vi "DMM6500.vi"(8 "error in (no error)":errorcluster) -> (0 "error in (out)":errorcluster)   [LabVIEW 2024, in "DMM6500.lvlib"]
doc: "This template is for the Queued Message Handler design pattern.\n\nThe Event Handling Loop generates messages based on user interface actions.\n\nThe Message Handling Loop processes messages generated by the Event Handling Loop, or by other messages. The messages are string values, so new messages can be added easily to the Message Cases case structure in the Message Handling Loop. Each message cluster can also provide an optional value for Message Data, which is a variant that can be converted to whatever message-specific data is required."
uses:
  DMM6500.lvlib
  controls/DMM6500 UI Data.ctl
  Settings/support/DAQ_Config.ctl
  PrivateControls/DMM6500_FGV_Queue_Control.ctl
  687c9c7c-8178-403c-bf7e-b93dd3f91936.vi
  21044260-a770-49ae-a215-1be9417de303.vi
  <instrlib>/Keithley DMM6500 DAQ6500 Series/Public/Data/Read (Multiple Points).vi
  <vilib>/Utility/error.llb/Error Cluster From Error Code.vi
  <vilib>/ErrorRing/Error Ring.xnode
  support/Message Queue/DMM6500 Message Queue.lvlib
  support/User Event - Stop/DMM6500 User Event - Stop.lvlib
  <instrlib>/Keithley DMM6500 DAQ6500 Series/Keithley DMM6500 DAQ6500 Series.lvlib
  Launcher/Launcher_DTU.lvlib
  Settings/Setting_Screen.lvlib
  <instrlib>/Keithley DMM6500 DAQ6500 Series/Public/Data/Read (Single Point).vi
panel:
  out "status":bool
  in  "Scan Count (2)":u32=5
  in  "Config":string
  in  "DUT":string
  in  "Scan Count (1)":u32=5
  in  "DMM6500":refnum<visa-resource-name>="USB0::0x05E6::0x6510::04596852::INSTR"
  out "Data":dbl[](array[numeric])
  in  "Channel List(\"\")":string
  in  "Function":i32(ring) items=["Voltage DC", "Voltage AC", "Current DC", "Current AC", "Resistance", "4-wire Resistance", "Diode", "Capacitance", "Temperature", "Continuity", "Frequency", "Period", "Voltage Ratio", "Digitize Voltage", "Digitize Current"]
  out "queue name 2":string
  out "queue name":string
  out "Display <Replace Me>":string
  in  "Measure":bool
  in  "Do Something <Replace Me>":bool
  in  "Exit":bool
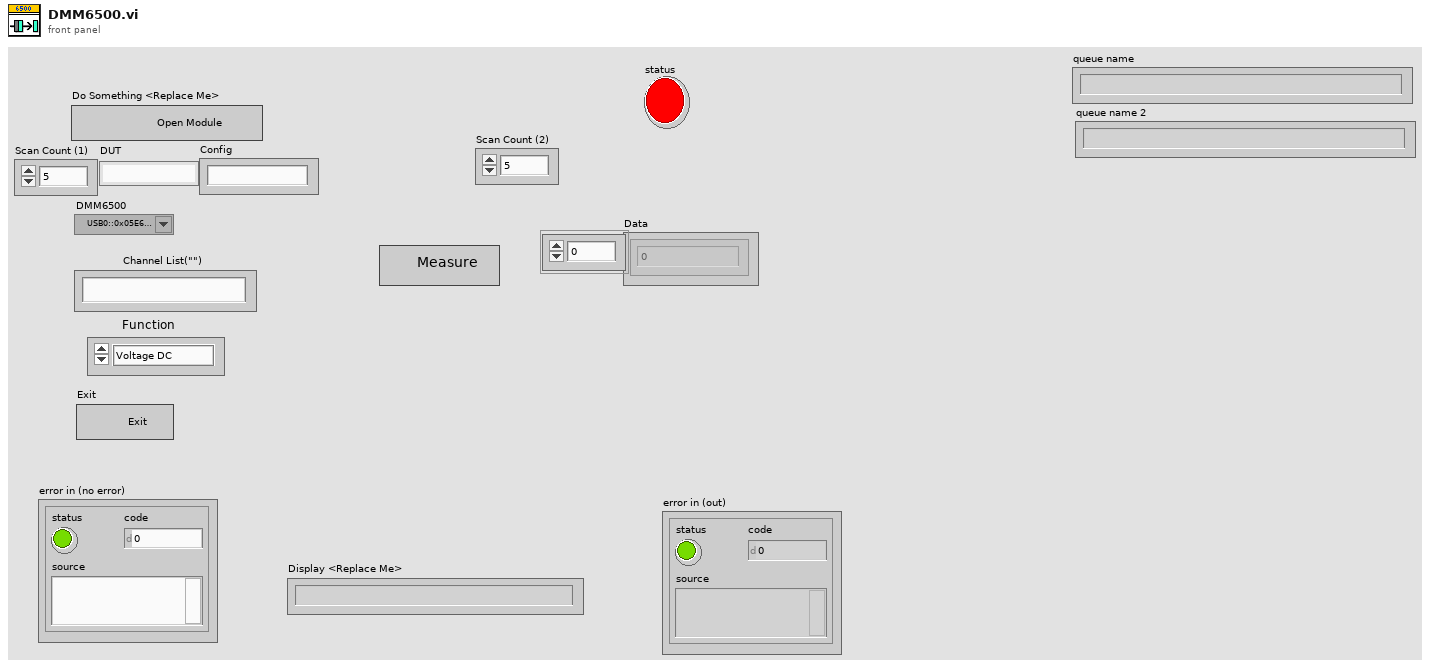
[diagram p1: front panel]
types:
  T1 = typedef "DMM6500.lvlib/DMM6500 UI Data.ctl" = cluster{"Config":string, "VISA":refnum<visa-resource-name>, "Function":i32, "Channel List(\"\")":string, "VISA resource name":refnum<visa-resource-name>, "Pseudo Card (0:No pseudocard)":i32, "Slot Number (0: slot1)":i32, "queue in":refnum<queue>, "DUT":string, "notifier out":refnum<notifier>}
  T2 = typedef "DMM6500.lvlib/DMM6500_FGV_Queue_Control.ctl" = enum16{"Release", "Get", "Set"}
  T3 = typedef "DMM6500.lvlib/DMM6500 Message Queue.lvlib/DMM6500_All Message Queues.ctl" = cluster{"UI":refnum<queue>, "QSM":refnum<queue>}
  T4 = cluster{"Message":string, "Message Data":variant}
  T5 = cluster{"Baud Rate":u32, "Flow Control":u16, "Parity":u16, "Stop Bits":u16, "Data Bits":u16}
  T6 = enum16{"Read", "Write", "All_sections", "All_values", "Remove key&section"}
  T7 = typedef "Setting_Screen.lvlib/DAQ_Config.ctl" = cluster{"AUTO RANGE":bool, "CHANNEL LIST":string, "SELECT Card":u16, "SELECT SLOT":u16, "Function":i32}
  T8 = cluster{"Function":i32, "Channel List(\"\")":string}
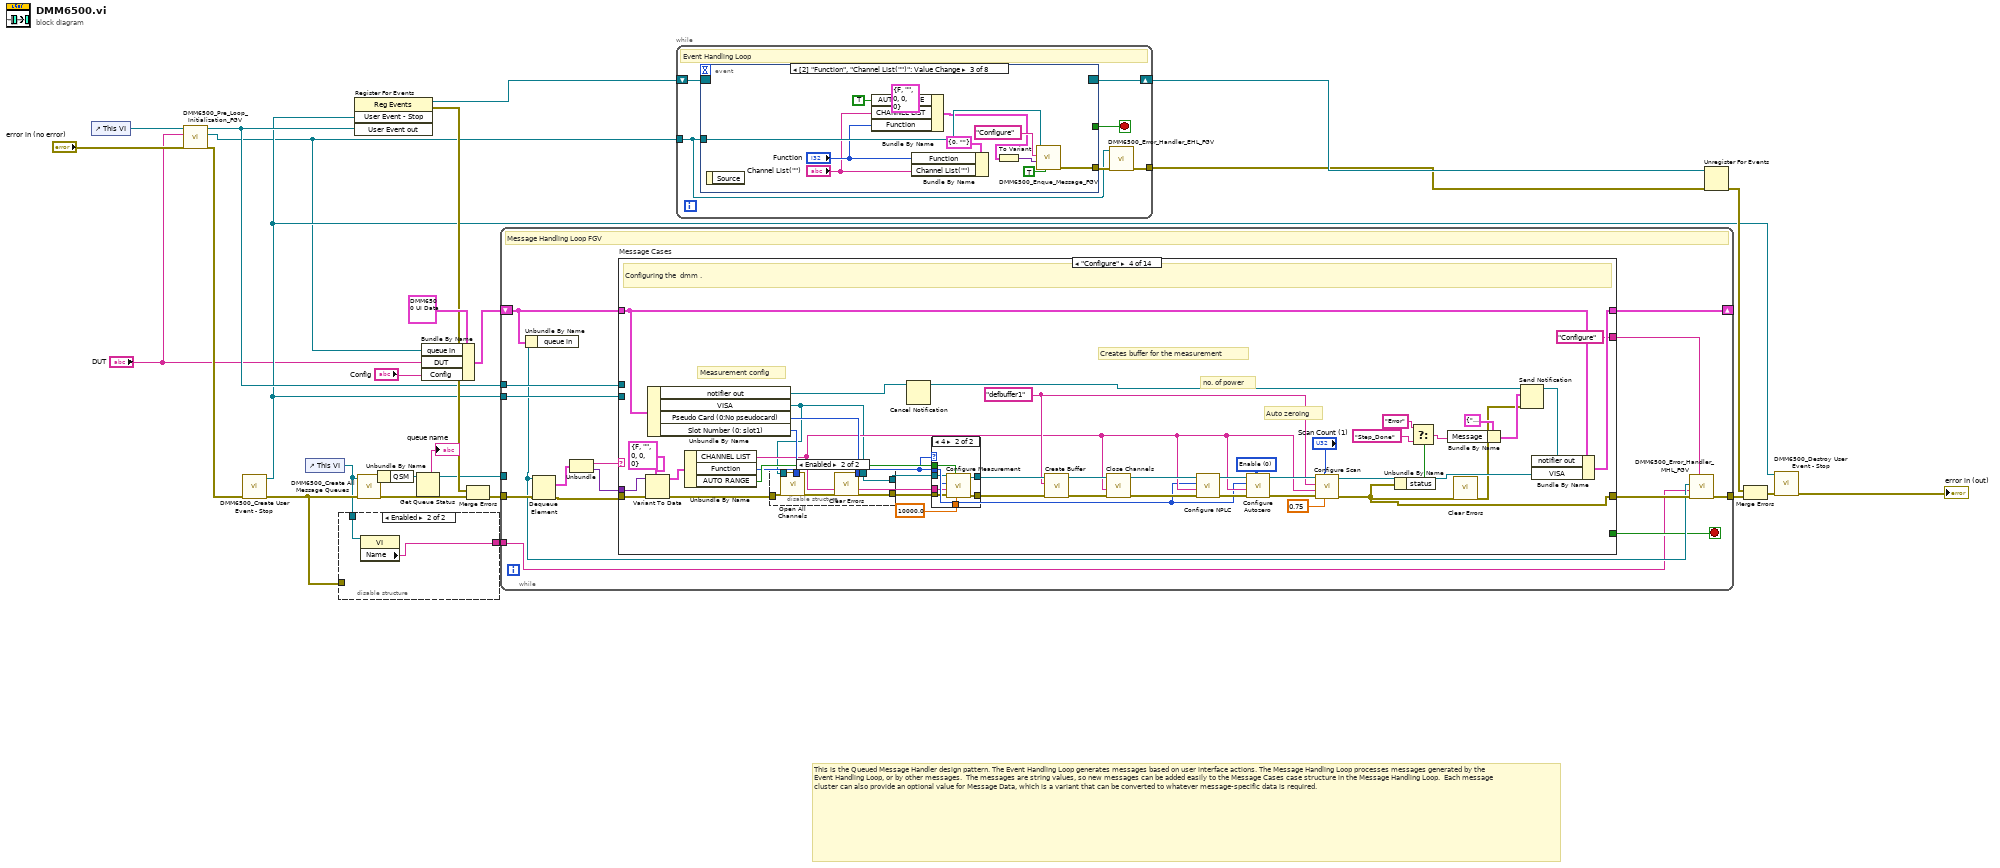
[diagram p0: block diagram]
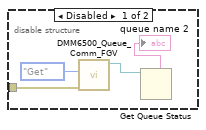
[diagram p2: hidden frame]
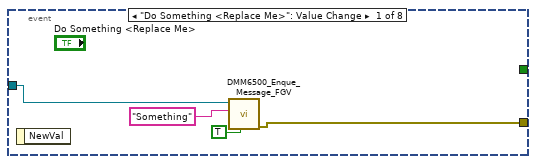
[diagram p3: hidden frame]
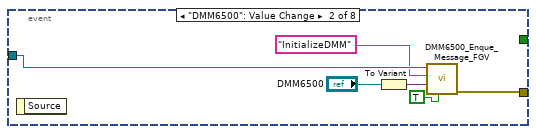
[diagram p4: hidden frame]
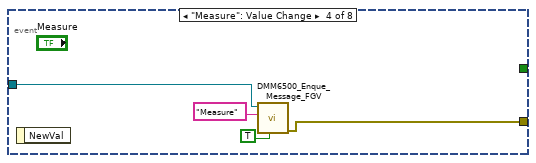
[diagram p5: hidden frame]
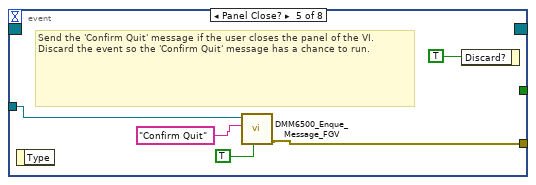
[diagram p6: hidden frame]
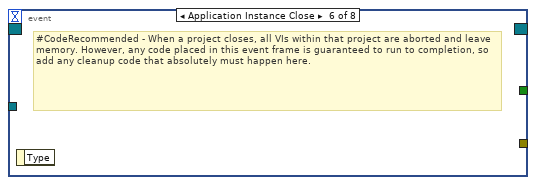
[diagram p7: hidden frame]
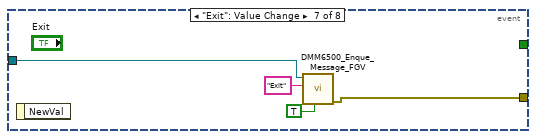
[diagram p8: hidden frame]
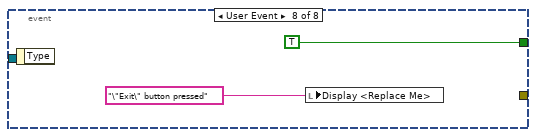
[diagram p9: hidden frame]
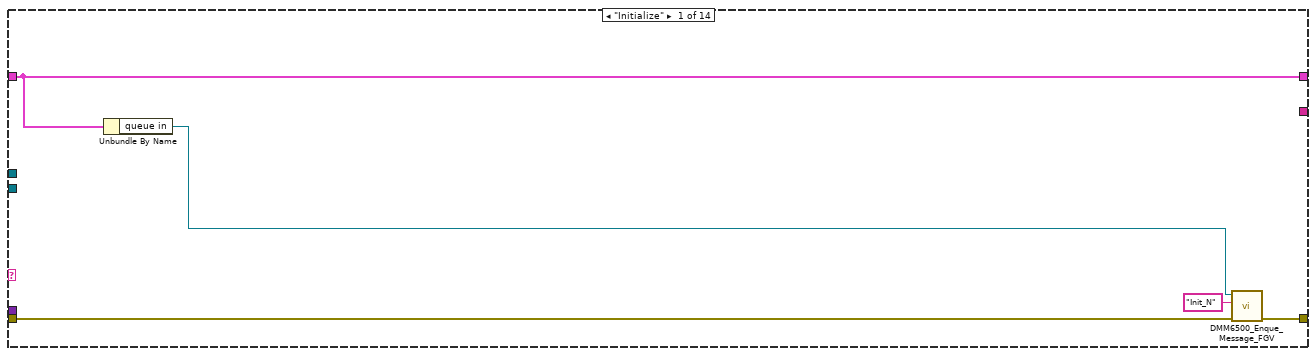
[diagram p10: hidden frame]
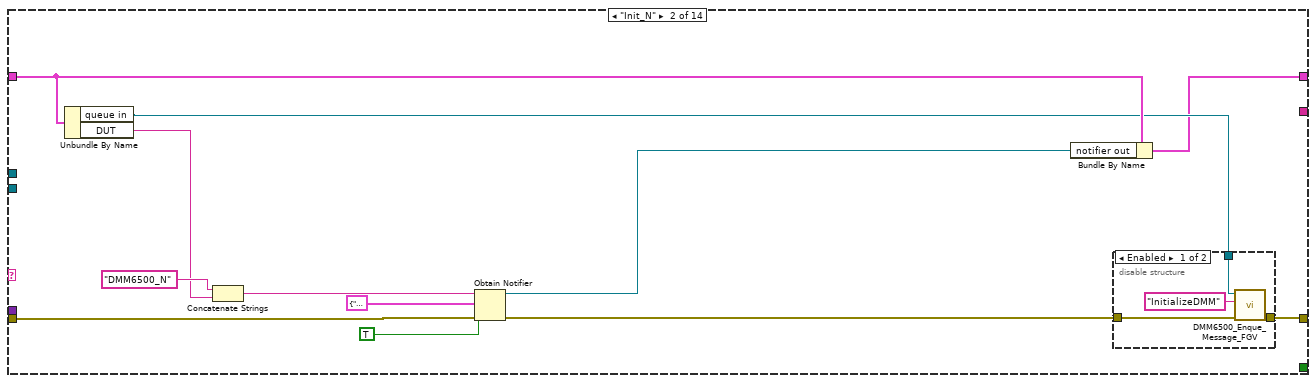
[diagram p11: hidden frame]
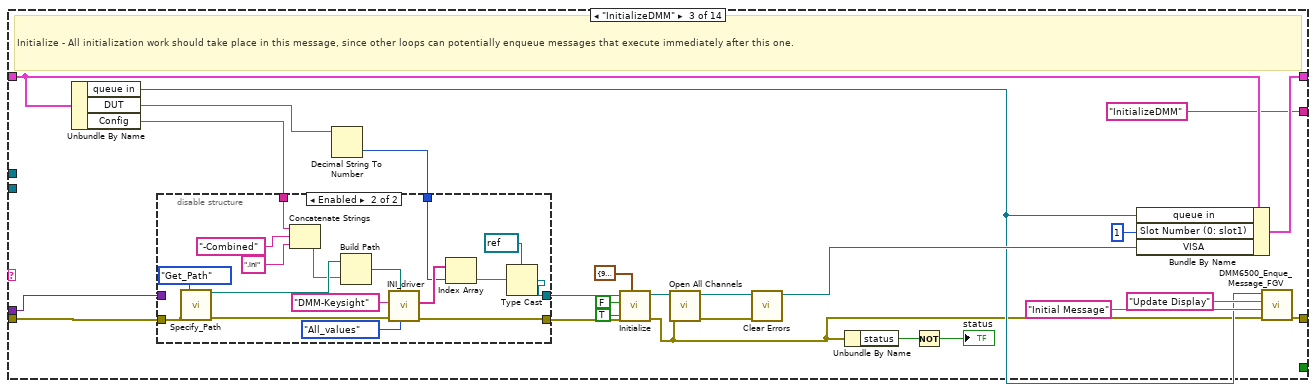
[diagram p13: hidden frame]
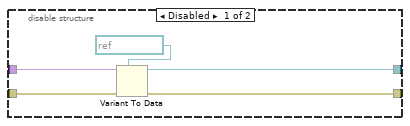
[diagram p14: hidden frame]
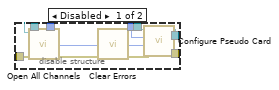
[diagram p15: hidden frame]
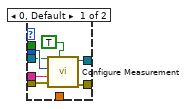
[diagram p16: hidden frame]
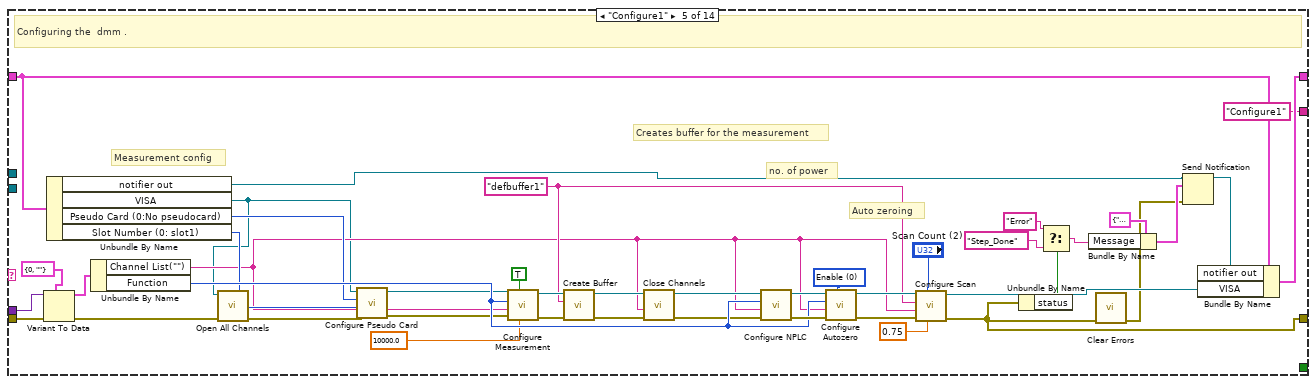
[diagram p17: hidden frame]
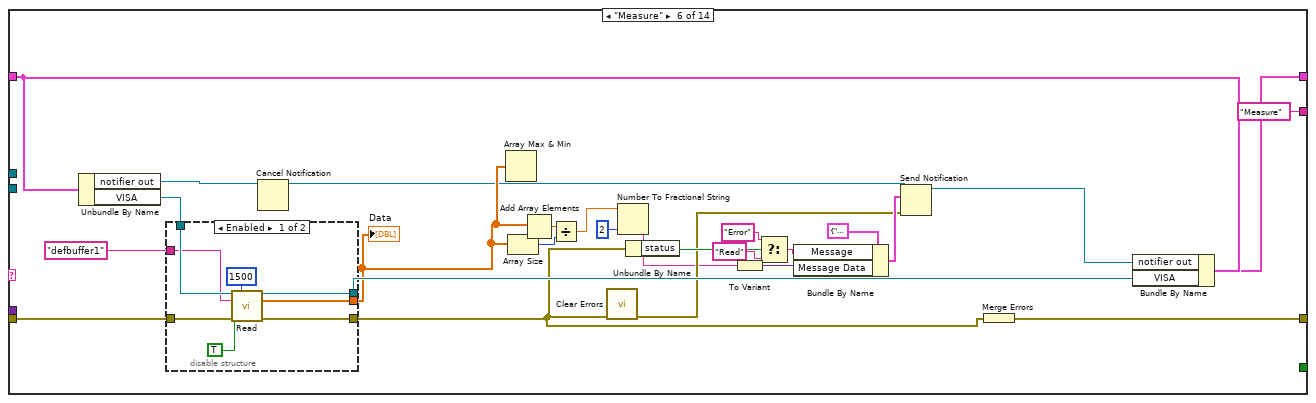
[diagram p18: hidden frame]
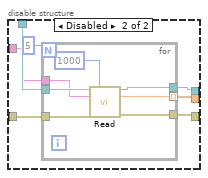
[diagram p19: hidden frame]
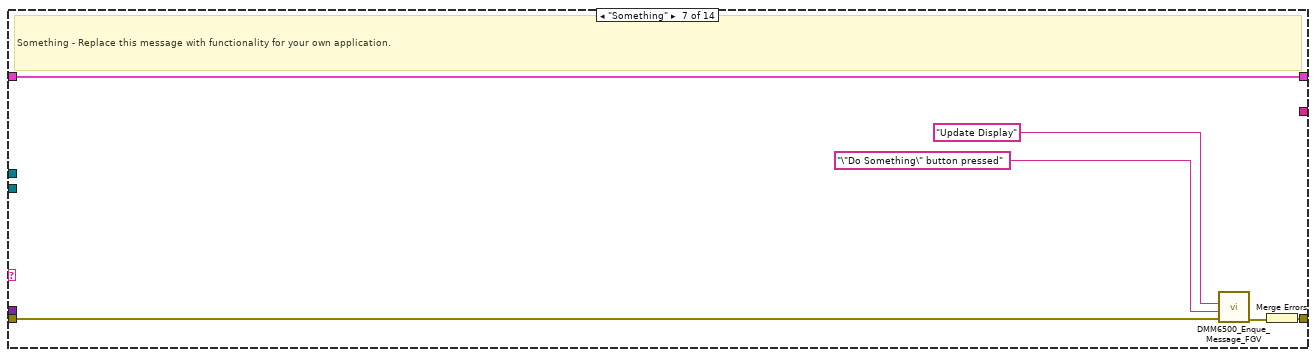
[diagram p20: hidden frame]
diagram:
  # "This is the Queued Message Handler design pattern. The Event Handling Loop generates messages based on user interface actions. The Message Handling Loop processes messages generated by the Event Handling Loop, or by other messages.  The messages are string values, so new messages can be added easily to the Message Cases case structure in the Message Handling Loop.  Each message cluster can also provide an optional value for Message Data, which is a variant that can be converted to whatever message-specific data is required."
  n1 = control-ref of="This VI"() -> (w15:refnum<vi>)
  n2 = call "DMM6500_Pre_Loop_Initialization_FGV.vi"("error in (no error)"="error in (no error)", "DUT"="DUT", "VI in"=w15) -> ("error out"=w13:errorcluster, "queue out"=w5:refnum<queue>, "User Event out"=w8:refnum<user-event>)  [unwired: 6 in]
  n3 = call "DMM6500_Create User Event - Stop.vi"("error in (no error)"=w13) -> ("error out"=w9:errorcluster, "User Event - Stop"=w7:refnum<user-event>)  [unwired: 9 in]
  n4 = control-ref of="This VI"() -> (w2:refnum<vi>)
  n5 = disable-structure shown="Enabled" {
    disable-tunnel: w9 -> [w31 _]
    disable-tunnel: w2 -> [_ w33]
    disable-tunnel: [_ w32] -> w1
    frame Disabled {
      n6 = call "DMM6500_Queue_Comm_FGV.vi"("error in (no error)"=w31, "Enum"=DMM6500_FGV_Queue_Control."Get") -> ("queue Out"=w29:refnum<queue>)  [unwired: 8 in, 1 out]
      n7 = Get Queue Status(queue=w29) -> (queue name=→"queue name 2":string)  [unwired: 2 in, 7 out]
    }
    frame Enabled {
      n8 = property class="VI"(reference=w33) -> ("Name"=w32:string)  [unwired: 1 in, 2 out]
    }
  }
  n9 = register-events(w7, w8) -> (reference out=w18:refnum<event-registration>, error out=w16:errorcluster)  [unwired: 2 in]
  n10 = call "DMM6500_Create All Message Queues.vi"("error in (no error)"=w9, "This VI"=w2) -> ("error out"=w27:errorcluster, "Message Queues out"=w26:T3)  [unwired: 8 in]
  n11 = Unbundle By Name(w26) -> ("QSM"=w24:refnum<queue>)
  n12 = Get Queue Status(queue=w24) -> (queue out=w11:refnum<queue>, queue name=→"queue name":string)  [unwired: 2 in, 6 out]
  n13 = Bundle By Name(cluster=T1 {"Config"="", "VISA"="", "Function"=0, "Channel List(\"\")"="", "VISA resource name"="USB0::0x05E6::0x6510::04596852::INSTR", "Pseudo Card (0:No pseudocard)"=0, "Slot Number (0: slot1)"=0, "queue in"=refnum, "DUT"="", "notifier out"=refnum} ("Data Cluster"), "queue in"=w5, "DUT"="DUT", "Config"="Config") -> (w6:T1)
  n14 = Merge Errors(w16, w27) -> (w17:errorcluster)
  n15 = while {
    tunnel: w11 -> [_]
    shift-right: [w48] -> _
    shift-left: w6 -> [w41]
    tunnel: w8 -> [w47]
    tunnel: w17 -> [w43]
    tunnel: [w45] -> w25
    tunnel: w7 -> [w44]
    tunnel: w1 -> [w35]
    stop <- w36 stop-if-true
    # "Message Handling Loop FGV"
    n16 = Unbundle By Name(w41) -> ("queue in"=w37:refnum<queue>)
    n17 = Dequeue Element(queue=w37, error in (no error)=w43) -> (element=w40:T4, error out=w42:errorcluster)  [unwired: 1 in, 2 out]
    n18 = Unbundle(w40) -> ("Message"=w39:string, "Message Data"=w38:variant)
    n19 = case "Message Cases" shown="\"Configure\"" w39 {
      selector: w39 -> [_ _ _ _ _ _ _ _ _ _ _ _ _ w363]
      tunnel: w42 -> [w53 w58 w83 w145 w215 w256 w279 w285 w295 w311 w326 w345 w358 _]
      tunnel: [w52 w65 w93 w120 w189 w242 w283 w289 w296 w300 w316 w347 w349 w364] -> w46
      tunnel: w41 -> [w50 w64 w90 w159 w230 w255 w284 w290 w297 w309 w322 w342 w353 w365]
      tunnel: [w50 w55 w94 w148 w218 w252 w284 w290 w297 w309 w322 w342 w353 w365] -> w48
      tunnel: [_ _ _ _ _ _ _ _ _ _ _ _ TRUE _] -> w36
      tunnel: w38 -> [_ _ w84 w146 w216 _ _ _ w294 _ w325 _ _ _]
      tunnel: w47 -> [_ _ _ _ _ _ _ _ _ _ _ _ w360 _]
      tunnel: w44 -> [_ _ _ _ _ _ _ _ _ _ _ _ w356 _]
      tunnel: [_ _ "InitializeDMM" "Configure" "Configure1" "Measure" _ _ _ _ "Error" _ _ _] -> w34
      frame "Initialize" {
        n20 = Unbundle By Name(w50) -> ("queue in"=w49:refnum<queue>)
        n21 = call "DMM6500_Enque_Message_FGV.vi"("error in (no error)"=w53, "Message"="Init_N", "queue In"=w49) -> ("error out"=w52:errorcluster)  [unwired: 8 in]
      }
      frame "Init_N" {
        n22 = Unbundle By Name(w64) -> ("queue in"=w63:refnum<queue>, "DUT"=w56:string)
        n23 = Concatenate Strings("DMM6500_N", w56) -> (w61:string)
        n24 = Obtain Notifier(name (unnamed)=w61, notification data type=T4 {"Message"="", "Message Data"=variant} ("notification"), create if not found? (T)=TRUE, error in (no error)=w58) -> (notifier out=w54:refnum<notifier>, error out=w57:errorcluster)  [unwired: 1 out]
        n25 = Bundle By Name(cluster=w64, "notifier out"=w54) -> (w55:T1)
        n26 = disable-structure shown="Enabled" {
          disable-tunnel: [w68 w70] -> w65
          disable-tunnel: w63 -> [w67 _]
          disable-tunnel: w57 -> [w66 w70]
          frame Enabled {
            n27 = call "DMM6500_Enque_Message_FGV.vi"("error in (no error)"=w66, "Message"="InitializeDMM", "queue In"=w67) -> ("error out"=w68:errorcluster)  [unwired: 8 in]
          }
          frame Disabled {
          }
        }
      }
      frame "InitializeDMM" {
        # "Initialize - All initialization work should take place in this message, since other loops can potentially enqueue messages that execute immediately after this one."
        n28 = Unbundle By Name(w90) -> ("queue in"=w86:refnum<queue>, "DUT"=w81:string, "Config"=w85:string)
        n29 = Decimal String To Number(string=w81) -> (number=w80:i32)  [unwired: 2 in, 1 out]
        n30 = disable-structure shown="Enabled" {
          disable-tunnel: w83 -> [w99 w104]
          disable-tunnel: [w98 w102] -> w82
          disable-tunnel: w84 -> [w97 _]
          disable-tunnel: [w95 w103] -> w79
          disable-tunnel: w85 -> [_ w101]
          disable-tunnel: w80 -> [_ w100]
          frame Disabled {
            n31 = Variant To Data(error in=w99, type=refnum<visa-resource-name> "COM27" ("VISA resource name"), Variant=w97) -> (data=w95:refnum<visa-resource-name>, error out=w98:errorcluster)
          }
          frame Enabled {
            n32 = call "Specify_Path.vi"("Path_Enum"=enum16{"Find_Path", "Get_Path"}."Get_Path", "error in (no error)"=w104) -> ("Configurations"=w113:path, "error out"=w109:errorcluster)  [unwired: 6 in, 6 out]
            n33 = Concatenate Strings(w101, "-Combined" ("string"), ".ini" ("string")) -> (w112:string)
            n34 = Build Path(base path=w113, name or relative path=w112) -> (appended path=w111:path)
            n35 = call "INI_driver.vi"("Enum"=T6."All_values", "instrument file path"=w111, "error in (no error)"=w109, "Section"="DMM-Keysight") -> ("error out"=w102:errorcluster, "Values out"=w107:string[])  [unwired: 4 in, 2 out]
            n36 = Index Array(array=w107, index=w100) -> (element=w106:string)
            n37 = Type Cast(type=refnum<visa-resource-name> refnum ("VISA resource name"), x=w106) -> (*(type *) &x=w103:refnum<visa-resource-name>)
          }
        }
        n38 = call <instrlib>:"Initialize.vi"("Serial Configuration"=T5 {"Baud Rate"=9600, "Flow Control"=0, "Parity"=0, "Stop Bits"=10, "Data Bits"=8}, "error in (no error)"=w82, "Reset (True)"=TRUE, "ID Query (True)"=FALSE, "VISA resource name"=w79) -> ("error out"=w71:errorcluster, "VISA resource name out"=w88:refnum<visa-resource-name>)  [unwired: 5 in]
        n39 = call <instrlib>:"Open All Channels.vi"("error in (no error)"=w71, "VISA resource name"=w88) -> ("error out"=w74:errorcluster, "VISA resource name out"=w87:refnum<visa-resource-name>)  [unwired: 8 in]
        n40 = call <vilib>:"Clear Errors.vi"("error in (no error)"=w74) -> ()  [unwired: 5 in, 2 out]
        n41 = Unbundle By Name(w71) -> ("status"=w73:bool)
        n42 = Not(x=w73) -> (.not. x?=→"status":bool)
        n43 = Bundle By Name(cluster=w90, "queue in"=w86, "Slot Number (0: slot1)"=1, "VISA"=w87) -> (w94:T1)
        n44 = call "DMM6500_Enque_Message_FGV.vi"("error in (no error)"=w71, "Message Data"="Initial Message" ("Initial Message"), "Message"="Update Display", "queue In"=w86) -> ("error out"=w93:errorcluster)  [unwired: 7 in]
      }
      frame "Configure" {
        w151 = u32 0 items=["Enable", "Disable", "Once"] ("Auto Zero (0: Enable)")
        w150 = "defbuffer1" ("Buffer Name (\"\")")
        # "Auto zeroing"
        # "no. of power"
        # "Creates buffer for the measurement"
        # "Measurement config"
        # "Configuring the  dmm ."
        n45 = Variant To Data(error in=w145, type=T7 {"AUTO RANGE"=FALSE, "CHANNEL LIST"="", "SELECT Card"=0, "SELECT SLOT"=0, "Function"=0} ("DAQ_Config"), Variant=w146) -> (data=w144:T7, error out=w143:errorcluster)
        n46 = Unbundle By Name(w159) -> ("notifier out"=w128:refnum<notifier>, "VISA"=w118:refnum<visa-resource-name>, "Pseudo Card (0:No pseudocard)"=w141:i32, "Slot Number (0: slot1)"=w140:i32)
        n47 = Unbundle By Name(w144) -> ("CHANNEL LIST"=w135:string, "Function"=w121:i32, "AUTO RANGE"=w122:bool)
        n48 = disable-structure shown="Enabled" {
          disable-tunnel: w143 -> [w167 w171]
          disable-tunnel: [w166 w172] -> w142
          disable-tunnel: w141 -> [w165 _]
          disable-tunnel: w140 -> [w164 _]
          disable-tunnel: [w163 w168] -> w139
          disable-tunnel: w118 -> [w161 w172]
          disable-tunnel: w118 -> [_ w169]
          frame Disabled {
            n49 = call <instrlib>:"Open All Channels.vi"("error in (no error)"=w167, "VISA resource name"=w161) -> ("error out"=w162:errorcluster)  [unwired: 8 in, 1 out]
            n50 = call <vilib>:"Clear Errors.vi"("error in (no error)"=w162) -> ("error out"=w160:errorcluster)  [unwired: 5 in, 1 out]
            n51 = call <instrlib>:"Configure Pseudo Card.vi"("error in (no error)"=w160, "Slot Number (0: slot1)"=w164, "Pseudo Card (0:No pseudocard)"=w165, "VISA resource name"=w161) -> ("error out"=w163:errorcluster, "VISA resource name out"=w166:refnum<visa-resource-name>)  [unwired: 6 in]
          }
          frame Enabled {
            n52 = call <instrlib>:"Open All Channels.vi"("error in (no error)"=w171, "VISA resource name"=w169) -> ("error out"=w170:errorcluster)  [unwired: 8 in, 1 out]
            n53 = call <vilib>:"Clear Errors.vi"("error in (no error)"=w170) -> ("error out"=w168:errorcluster)  [unwired: 5 in, 1 out]
          }
        }
        n54 = Cancel Notification(0:w128) -> (8:w117:refnum<notifier>)  [unwired: 1 in, 2 out]
        n55 = case shown="4" w121 {
          tunnel: [w179 w187] -> w158
          tunnel: [w178 w186] -> w157
          tunnel: w121 -> [w177 w185]
          tunnel: w142 -> [w176 w184]
          tunnel: w139 -> [w175 w183]
          tunnel: w135 -> [w174 w182]
          tunnel: 10000.0 ("Manual Range (1)") -> [_ w181]
          tunnel: w122 -> [_ w180]
          frame 0, Default {
            n56 = call <instrlib>:"Configure Measurement.vi"("Auto Range (T: Enable)"=TRUE, "error in (no error)"=w175, "Channel List(\"\")"=w174, "Function (0: Voltage DC)"=w177, "VISA resource name"=w176) -> ("error out"=w179:errorcluster, "VISA resource name out"=w178:refnum<visa-resource-name>)  [unwired: 5 in]
          }
          frame 4 {
            n57 = call <instrlib>:"Configure Measurement.vi"("Manual Range (1)"=w181, "Auto Range (T: Enable)"=w180, "error in (no error)"=w183, "Channel List(\"\")"=w182, "Function (0: Voltage DC)"=w185, "VISA resource name"=w184) -> ("error out"=w187:errorcluster, "VISA resource name out"=w186:refnum<visa-resource-name>)  [unwired: 4 in]
          }
        }
        n58 = call <instrlib>:"Create Buffer.vi"("error in (no error)"=w158, "Buffer Name (\"\")"=w150, "VISA resource name"=w157) -> ("error out"=w154:errorcluster, "VISA resource name out"=w137:refnum<visa-resource-name>)  [unwired: 7 in]
        n59 = call <instrlib>:"Close Channels.vi"("error in (no error)"=w154, "Channel List(\"\")"=w135, "VISA resource name"=w137) -> ("error out"=w138:errorcluster, "VISA resource name out"=w136:refnum<visa-resource-name>)  [unwired: 7 in]
        n60 = call <instrlib>:"Configure NPLC.vi"("error in (no error)"=w138, "Channel List(\"\")"=w135, "Function (0: Voltage DC)"=w121, "VISA resource name"=w136) -> ("error out"=w153:errorcluster, "VISA resource name out"=w152:refnum<visa-resource-name>)  [unwired: 6 in]
        n61 = call <instrlib>:"Configure Autozero.vi"("Auto Zero (0: Enable)"=w151, "error in (no error)"=w153, "Channel List(\"\")"=w135, "Function (0: Voltage DC)"=w121, "VISA resource name"=w152) -> ("error out"=w156:errorcluster, "VISA resource name out"=w155:refnum<visa-resource-name>)  [unwired: 5 in]
        n62 = call <instrlib>:"Configure Scan.vi"("Delay Seconds (0 s)"=0.75, "Scan Count (1)"="Scan Count (1)", "error in (no error)"=w156, "Channel List(\"\")"=w135, "Reading Buffer (\"\")"=w150, "VISA resource name"=w155) -> ("error out"=w120:errorcluster, "VISA resource name out"=w147:refnum<visa-resource-name>)  [unwired: 4 in]
        n63 = Unbundle By Name(w120) -> ("status"=w129:bool)
        n64 = Select(t="Error" ("f"), s=w129, f="Step_Done" ("Message")) -> (s? t:f=w133:string)
        n65 = Bundle By Name(cluster=T4 {"Message"="", "Message Data"=variant} ("notification"), "Message"=w133) -> (w127:T4)
        n66 = call <vilib>:"Clear Errors.vi"("error in (no error)"=w120) -> ("error out"=w125:errorcluster)  [unwired: 5 in, 1 out]
        n67 = Send Notification(notification=w127, notifier=w117, error in (no error)=w125) -> (notifier out=w126:refnum<notifier>)  [unwired: 1 out]
        n68 = Bundle By Name(cluster=w159, "notifier out"=w126, "VISA"=w147) -> (w148:T1)
      }
      frame "Configure1" {
        w221 = u32 0 items=["Enable", "Disable", "Once"] ("Auto Zero (0: Enable)")
        w220 = "defbuffer1" ("Buffer Name (\"\")")
        # "Auto zeroing"
        # "no. of power"
        # "Creates buffer for the measurement"
        # "Measurement config"
        # "Configuring the  dmm ."
        n69 = Variant To Data(error in=w215, type=T8 {"Function"=0, "Channel List(\"\")"=""}, Variant=w216) -> (data=w214:T8, error out=w212:errorcluster)
        n70 = Unbundle By Name(w230) -> ("notifier out"=w195:refnum<notifier>, "VISA"=w202:refnum<visa-resource-name>, "Pseudo Card (0:No pseudocard)"=w210:i32, "Slot Number (0: slot1)"=w209:i32)
        n71 = Unbundle By Name(w214) -> ("Channel List(\"\")"=w204:string, "Function"=w213:i32)
        n72 = call <instrlib>:"Open All Channels.vi"("error in (no error)"=w212, "VISA resource name"=w202) -> ("error out"=w203:errorcluster)  [unwired: 8 in, 1 out]
        n73 = call <instrlib>:"Configure Pseudo Card.vi"("error in (no error)"=w203, "Slot Number (0: slot1)"=w209, "Pseudo Card (0:No pseudocard)"=w210, "VISA resource name"=w202) -> ("error out"=w208:errorcluster, "VISA resource name out"=w211:refnum<visa-resource-name>)  [unwired: 6 in]
        n74 = call <instrlib>:"Configure Measurement.vi"("Manual Range (1)"=10000.0, "Auto Range (T: Enable)"=TRUE, "error in (no error)"=w208, "Channel List(\"\")"=w204, "Function (0: Voltage DC)"=w213, "VISA resource name"=w211) -> ("error out"=w228:errorcluster, "VISA resource name out"=w227:refnum<visa-resource-name>)  [unwired: 4 in]
        n75 = call <instrlib>:"Create Buffer.vi"("error in (no error)"=w228, "Buffer Name (\"\")"=w220, "VISA resource name"=w227) -> ("error out"=w224:errorcluster, "VISA resource name out"=w206:refnum<visa-resource-name>)  [unwired: 7 in]
        n76 = call <instrlib>:"Close Channels.vi"("error in (no error)"=w224, "Channel List(\"\")"=w204, "VISA resource name"=w206) -> ("error out"=w207:errorcluster, "VISA resource name out"=w205:refnum<visa-resource-name>)  [unwired: 7 in]
        n77 = call <instrlib>:"Configure NPLC.vi"("error in (no error)"=w207, "Channel List(\"\")"=w204, "Function (0: Voltage DC)"=w213, "VISA resource name"=w205) -> ("error out"=w223:errorcluster, "VISA resource name out"=w222:refnum<visa-resource-name>)  [unwired: 6 in]
        n78 = call <instrlib>:"Configure Autozero.vi"("Auto Zero (0: Enable)"=w221, "error in (no error)"=w223, "Channel List(\"\")"=w204, "Function (0: Voltage DC)"=w213, "VISA resource name"=w222) -> ("error out"=w226:errorcluster, "VISA resource name out"=w225:refnum<visa-resource-name>)  [unwired: 5 in]
        n79 = call <instrlib>:"Configure Scan.vi"("Delay Seconds (0 s)"=0.75, "Scan Count (1)"="Scan Count (2)", "error in (no error)"=w226, "Channel List(\"\")"=w204, "Reading Buffer (\"\")"=w220, "VISA resource name"=w225) -> ("error out"=w189:errorcluster, "VISA resource name out"=w217:refnum<visa-resource-name>)  [unwired: 4 in]
        n80 = Unbundle By Name(w189) -> ("status"=w196:bool)
        n81 = Select(t="Error" ("f"), s=w196, f="Step_Done" ("Message")) -> (s? t:f=w200:string)
        n82 = Bundle By Name(cluster=T4 {"Message"="", "Message Data"=variant} ("notification"), "Message"=w200) -> (w194:T4)
        n83 = call <vilib>:"Clear Errors.vi"("error in (no error)"=w189) -> ("error out"=w192:errorcluster)  [unwired: 5 in, 1 out]
        n84 = Send Notification(notification=w194, notifier=w195, error in (no error)=w192) -> (notifier out=w193:refnum<notifier>)  [unwired: 1 out]
        n85 = Bundle By Name(cluster=w230, "notifier out"=w193, "VISA"=w217) -> (w218:T1)
      }
      frame "Measure" {
        n86 = Unbundle By Name(w255) -> ("notifier out"=w232:refnum<notifier>, "VISA"=w254:refnum<visa-resource-name>)
        n87 = disable-structure shown="Enabled" {
          disable-tunnel: w256 -> [w264 w271]
          disable-tunnel: w254 -> [w263 w267]
          disable-tunnel: "defbuffer1" ("Buffer Name (\"\")") -> [w262 w266]
          disable-tunnel: [w261 w268] -> w251
          disable-tunnel: [w260 w269] -> w236
          disable-tunnel: [w259 w270] -> w234
          frame Enabled {
            n88 = call-poly <instrlib>:"Read.vi"("VISA resource name"=w263, "Timeout (10000 ms)"=1500, "Buffer Name (\"\")"=w262, "Clear Buffer (No)"=TRUE, "error in (no error)"=w264) -> ("VISA resource name out"=w261:refnum<visa-resource-name>, "Measurements"=w260:dbl[], "error out"=w259:errorcluster)  [unwired: 8 in]
          }
          frame Disabled {
            n89 = for {
              N: 5 -> [_]
              tunnel: w271 -> [w278]
              tunnel: [w277] -> w270
              tunnel: [w276] -> w269 mode=indexing
              tunnel: [w275] -> w268
              tunnel: w267 -> [w274]
              tunnel: w266 -> [w273]
              n90 = call-poly <instrlib>:"Read.vi"("VISA resource name"=w274, "Timeout (100000ms)"=u32 1000, "Buffer Name (\"\")"=w273, "error in (no error)"=w278) -> ("VISA resource name out"=w275:refnum<visa-resource-name>, "Measurement"=w276:dbl, "error out"=w277:errorcluster)  [unwired: 9 in]
            }
          }
        }
        "Data" <- w236
        n91 = Cancel Notification(0:w232) -> (8:w231:refnum<notifier>)  [unwired: 1 in, 2 out]
        n92 = Array Max & Min(array=w236) -> ()  [unwired: 4 out]
        n93 = Array Size(array=w236) -> (size(s)=w239:i32)
        n94 = Add Array Elements(numeric array=w236) -> (sum=w240:dbl)
        n95 = Divide(x=w240, y=w239) -> (x/y=w235:dbl)
        n96 = call <vilib>:"Clear Errors.vi"("error in (no error)"=w234) -> ("error out"=w243:errorcluster)  [unwired: 5 in, 1 out]
        n97 = Number To Fractional String(number=w235, precision (6)=i16 2) -> (F-format string=w237:string)  [unwired: 2 in]
        n98 = Unbundle By Name(w234) -> ("status"=w244:bool)
        n99 = To Variant(anything=w237) -> (Variant=w247:variant)
        n100 = Select(t="Error" ("f"), s=w244, f="Read" ("Message")) -> (s? t:f=w250:string)
        n101 = Bundle By Name(cluster=T4 {"Message"="", "Message Data"=variant} ("notification"), "Message"=w250, "Message Data"=w247) -> (w245:T4)
        n102 = Send Notification(notification=w245, notifier=w231, error in (no error)=w243) -> (notifier out=w241:refnum<notifier>)  [unwired: 1 out]
        n103 = Merge Errors(w234) -> (w242:errorcluster)
        n104 = Bundle By Name(cluster=w255, "notifier out"=w241, "VISA"=w251) -> (w252:T1)
      }
      frame "Something" {
        # "Something - Replace this message with functionality for your own application."
        n105 = call "DMM6500_Enque_Message_FGV.vi"("error in (no error)"=w279, "Message Data"="\"Do Something\" button pressed" ("\"Do Something\" button pressed"), "Message"="Update Display") -> ("error out"=w282:errorcluster)  [unwired: 8 in]
        n106 = Merge Errors(w282) -> (w283:errorcluster)
      }
      frame "Something Else" {
        # "Send string to \"Update Display\" message"
        # "#CodeNeeded - Perform whatever actions correspond to the \"Something Else\" message."
        # "Something Else - Replace this message with functionality for your own application."
        n107 = call "DMM6500_Enque_Message_FGV.vi"("error in (no error)"=w285, "Message Data"="\"Do Something Else\" button pressed" ("\"Do Something Else\" button pressed"), "Message"="Update Display") -> ("error out"=w288:errorcluster)  [unwired: 8 in]
        n108 = Merge Errors(w288) -> (w289:errorcluster)
      }
      frame "Update Display" {
        # "#CodeRecommended - If you wish to decouple the Message Handling Loop from your user interface, consider creating User Events (like the \"Stop\" event in this VI) to message the Event Handling Loop whenever the user interface needs updating."
        # "Update Display - Convert the message data to a string to display in the Data Display indicator."
        n109 = Variant To Data(error in=w295, type="", Variant=w294) -> (data=→"Display <Replace Me>":string, error out=w292:errorcluster)
        n110 = Merge Errors(w292) -> (w296:errorcluster)
      }
      frame "Reset" {
        n111 = Unbundle By Name(w309) -> ("VISA"=w298:refnum<visa-resource-name>, "queue in"=w299:refnum<queue>)
        n112 = call <instrlib>:"Clear Buffer.vi"("error in (no error)"=w311, "Buffer Name (\"\")"="defbuffer1" ("Buffer Name (\"\")"), "VISA resource name"=w298) -> ("error out"=w310:errorcluster)  [unwired: 7 in, 1 out]
        n113 = call <vilib>:"Clear Errors.vi"("error in (no error)"=w310) -> ("error out"=w307:errorcluster)  [unwired: 5 in, 1 out]
        n114 = call <instrlib>:"Reset.vi"("error in (no error)"=w307, "VISA resource name"=w298) -> ("error out"=w301:errorcluster)  [unwired: 8 in, 1 out]
        n115 = call <vilib>:"Clear Errors.vi"("error in (no error)"=w301) -> ("error out"=w300:errorcluster)  [unwired: 5 in, 1 out]
        n116 = call <instrlib>:"Close.vi"("error in (no error)"=w300, "VISA resource name"=w298) -> ("error out"=w306:errorcluster)  [unwired: 9 in]
        n117 = call "Stall Data Flow.vim"("value in"=w306, "milliseconds to wait"=u32 1000) -> ("value out"=w303:errorcluster)  [unwired: 1 out]
        n118 = Merge Errors(w303) -> (w304:errorcluster)
        n119 = call "DMM6500_Enque_Message_FGV.vi"("error in (no error)"=w304, "Message"="InitializeDMM", "queue In"=w299) -> ()  [unwired: 8 in, 1 out]
      }
      frame "Error" {
        # "Error - Display an error dialog. This message is sent by the \"Error Handler\" VIs at the end of other loops in this application."
        n120 = disable-structure shown="Enabled" {
          disable-tunnel: w326 -> [w335 w337]
          disable-tunnel: w325 -> [w334 _]
          disable-tunnel: [w331 w336] -> w324
          frame Disabled {
            n121 = Variant To Data(error in=w335, type=errorcluster {"status"=FALSE, "code"=0, "source"=""} ("error constant"), Variant=w334) -> (data=w332:errorcluster, error out=w331:errorcluster)
            n122 = call <vilib>:"Simple Error Handler.vi"("error in (no error)"=w332) -> ()  [unwired: 4 in, 5 out]
          }
          frame Enabled {
            n123 = call <vilib>:"Clear Errors.vi"("error in (no error)"=w337) -> ("error out"=w336:errorcluster)  [unwired: 5 in, 1 out]
          }
        }
        n124 = Unbundle By Name(w322) -> ("queue in"=w315:refnum<queue>, "VISA resource name"=w319:refnum<visa-resource-name>)
        n125 = disable-structure shown="Enabled" {
          disable-tunnel: w324 -> [w329 w330]
          disable-tunnel: [w328 w330] -> w323
          disable-tunnel: w319 -> [w327 _]
          frame Enabled {
            n126 = call <instrlib>:"Reset.vi"("error in (no error)"=w329, "VISA resource name"=w327) -> ("error out"=w328:errorcluster)  [unwired: 8 in, 1 out]
          }
          frame Disabled {
          }
        }
        n127 = call <vilib>:"Clear Errors.vi"("error in (no error)"=w323) -> ("error out"=w321:errorcluster)  [unwired: 5 in, 1 out]
        n128 = call <instrlib>:"Close.vi"("error in (no error)"=w321, "VISA resource name"=w319) -> ("error out"=w320:errorcluster)  [unwired: 9 in]
        n129 = call "Stall Data Flow.vim"("value in"=w320, "milliseconds to wait"=u32 300) -> ("value out"=w313:errorcluster)  [unwired: 1 out]
        n130 = Merge Errors(w313) -> (w317:errorcluster)
        n131 = call "DMM6500_Enque_Message_FGV.vi"("error in (no error)"=w317, "Message"="InitializeDMM", "queue In"=w315) -> ("error out"=w316:errorcluster)  [unwired: 8 in]
      }
      frame "Confirm Quit" {
        # "Confirm Quit - Message that can confirm whether or not the user wants to exit the application."
        n132 = Unbundle By Name(w342) -> ("queue in"=w341:refnum<queue>, "notifier out"=w339:refnum<notifier>)
        n133 = Release Notifier(notifier=w339, force destroy? (F)=FALSE, error in (no error)=w345) -> (error out=w340:errorcluster)  [unwired: 2 out]
        n134 = call "DMM6500_Enque_Message_FGV.vi"("Priority"=TRUE ("Priority Message? (F)"), "error in (no error)"=w340, "Message"="Exit", "queue In"=w341) -> ("error out"=w346:errorcluster)  [unwired: 7 in]
        n135 = Merge Errors(w346) -> (w347:errorcluster)
      }
      frame "Exit" {
        # "Exit - Exit the application."
        n136 = Unbundle By Name(w353) -> ("VISA"=w351:refnum<visa-resource-name>, "queue in"=w350:refnum<queue>)
        n137 = call "DMM6500_Queue_Comm_FGV.vi"("error in (no error)"=w358, "Enum"=DMM6500_FGV_Queue_Control."Release", "queue in"=w350) -> ("error Out"=w357:errorcluster)  [unwired: 7 in, 1 out]
        n138 = call <vilib>:"Clear Errors.vi"("error in (no error)"=w357) -> ("error out"=w348:errorcluster)  [unwired: 5 in, 1 out]
        n139 = call <instrlib>:"Close.vi"("error in (no error)"=w348, "VISA resource name"=w351) -> ("error out"=w352:errorcluster)  [unwired: 9 in]
        n140 = call "DMM6500_Fire User Event - Stop.vi"("User Event - Stop"=w356) -> ("error out"=w354:errorcluster)  [unwired: 10 in]
        n141 = call "DMM6500_Fire User Event - Stop.vi"("User Event - Stop"=w360) -> ("error out"=w355:errorcluster)  [unwired: 10 in]
        n142 = Merge Errors(w355, w354, w352) -> (w361:errorcluster)
        n143 = call <vilib>:"Clear Errors.vi"("error in (no error)"=w361) -> ("error out"=w349:errorcluster)  [unwired: 5 in, 1 out]
      }
      frame Default {
        # "'Default' case only runs if there is a message that isn't defined in any of the other cases.  Output a programming error."
        n144 = xnode "Error Ring"("parameter 0"=w363) -> ("error out"=w364:errorcluster)
      }
    }
    n145 = call "DMM6500_Error_Handler_MHL_FGV.vi"("Case"=w34, "error in (no error)"=w46, "VI_name"=w35, "queue In"=w37) -> ("error Out"=w45:errorcluster)  [unwired: 7 in]
  }
  n146 = while {
    shift-right: [w377] -> w21
    shift-left: w18 -> [w378]
    tunnel: [w374] -> w19
    tunnel: w5 -> [w373]
    stop <- w376 stop-if-true
    # "Event Handling Loop"
    n147 = event shown="[2] \"Function\", \"Channel List(\"\")\": Value Change" {
      selector: w378 -> [_ _ _ _ _ _ _ _]
      dyn-events: [_ _ _ _ _ _ _ _] -> w377
      timeout: _ -> [_ _ _ _ _ _ _ _]
      tunnel: [_ _ _ _ _ _ _ TRUE ("Discard?")] -> w376
      tunnel: [w381 w387 w398 w401 w407 _ w412 _] -> w375
      tunnel: w373 -> [w379 w386 w394 w400 w404 _ w409 _]
      event "Do Something <Replace Me>": Value Change {
        n148 = event-data() -> ()  [unwired: 1 in, 1 out]
        n149 = call "DMM6500_Enque_Message_FGV.vi"("Priority"=TRUE ("Priority Message? (F)"), "Message"="Something", "queue In"=w379) -> ("error out"=w381:errorcluster)  [unwired: 8 in]
      }
      event "DMM6500": Value Change {
        n150 = event-data() -> ()  [unwired: 1 in, 1 out]
        n151 = To Variant(anything="DMM6500") -> (Variant=w384:variant)
        n152 = call "DMM6500_Enque_Message_FGV.vi"("Priority"=TRUE ("Priority Message? (F)"), "Message Data"=w384, "Message"="InitializeDMM", "queue In"=w386) -> ("error out"=w387:errorcluster)  [unwired: 7 in]
      }
      event "Function", "Channel List(\"\")": Value Change {
        n153 = event-data() -> ()  [unwired: 1 in, 1 out]
        n154 = Bundle By Name(cluster=T7 {"AUTO RANGE"=FALSE, "CHANNEL LIST"="", "SELECT Card"=0, "SELECT SLOT"=0, "Function"=0} ("data"), "AUTO RANGE"=TRUE, "CHANNEL LIST"="Channel List(\"\")", "Function"="Function") -> (w389:T7)
        n155 = Bundle By Name(cluster=T8 {"Function"=0, "Channel List(\"\")"=""}, "Function"="Function", "Channel List(\"\")"="Channel List(\"\")") -> ()  [unwired: 1 out]
        n156 = To Variant(anything=w389) -> (Variant=w395:variant)
        n157 = call "DMM6500_Enque_Message_FGV.vi"("Priority"=TRUE ("Priority Message? (F)"), "Message Data"=w395, "Message"="Configure", "queue In"=w394) -> ("error out"=w398:errorcluster)  [unwired: 7 in]
      }
      event "Measure": Value Change {
        n158 = event-data() -> ()  [unwired: 1 in, 1 out]
        n159 = call "DMM6500_Enque_Message_FGV.vi"("Priority"=TRUE ("Priority Message? (F)"), "Message"="Measure", "queue In"=w400) -> ("error out"=w401:errorcluster)  [unwired: 8 in]
      }
      event Panel Close? {
        # "Send the 'Confirm Quit' message if the user closes the panel of the VI. Discard the event so the 'Confirm Quit' message has a chance to run."
        n160 = event-data() -> ()  [unwired: 1 in, 1 out]
        n161 = call "DMM6500_Enque_Message_FGV.vi"("Priority"=TRUE ("Priority Message? (F)"), "Message"="Confirm Quit", "queue In"=w404) -> ("error out"=w407:errorcluster)  [unwired: 8 in]
        n162 = event-data("Discard?"=TRUE) -> ()  [unwired: 1 in, 1 out]
      }
      event Application Instance Close {
        # "#CodeRecommended - When a project closes, all VIs within that project are aborted and leave memory. However, any code placed in this event frame is guaranteed to run to completion, so add any cleanup code that absolutely must happen here."
        n163 = event-data() -> ()  [unwired: 1 in, 1 out]
      }
      event "Exit": Value Change {
        n164 = event-data() -> ()  [unwired: 1 in, 1 out]
        n165 = call "DMM6500_Enque_Message_FGV.vi"("Priority"=TRUE ("Priority Message? (F)"), "Message"="Exit", "queue In"=w409) -> ("error out"=w412:errorcluster)  [unwired: 8 in]
      }
      event User Event {
        n166 = event-data() -> ()  [unwired: 1 in, 1 out]
        n167 = local write "Display <Replace Me>"("\"Exit\" button pressed" ("VI Stopped")) -> ()
      }
    }
    n168 = call "DMM6500_Error_Handler_EHL_FGV.vi"("error in (no error)"=w375, "queue In"=w373) -> ("error Out"=w374:errorcluster)  [unwired: 9 in]
  }
  n169 = Unregister For Events(event registration refnum=w21, error in=w19) -> (error out=w22:errorcluster)
  n170 = Merge Errors(w22, w25) -> (w23:errorcluster)
  n171 = call "DMM6500_Destroy User Event - Stop.vi"("error in (no error)"=w23, "User Event - Stop"=w7) -> ("error out"=→"error in (out)":errorcluster)  [unwired: 9 in]
